vi "Buffer-GUI-parameter-values.vi"(8 "error in":errorcluster, 10 "UI ref. in":refnum<data-value>, 11 "Data ref. in":refnum<data-value>) -> (0 "error IO":errorcluster, 2 "UI ref.":refnum<data-value>, 3 "Data ref.":refnum<data-value>)   [LabVIEW 2013, in "CameraVision.lvlib" / "CV-Main.lvclass"]
doc: "This function copies the current values of the GUI parameter controls to the parameter group objects, by using the front panel object control references and the parameter group data value references."
uses:
  CV-Main.lvclass
  UI/CV-UI.lvclass
  UI/CV-UI.lvclass/CV-UI.ctl
  Configuration/Configuration-parameters-gui.ctl
  CV-Main.lvclass/CV-Main.ctl
  Acquisition/Acquisition-parameters-gui.ctl
  Acquisition/Trigger-modes.ctl
  Acquisition/Exposure-modes.ctl
  Correction/Correction-parameters-gui.ctl
  Correction/Smoothing.ctl
  Correction/Background-correction.ctl
  Analysis/Analysis-parameters-gui.ctl
  Temperature/Temperature-parameters-gui.ctl
  Mapping/Mapping-parameters-gui.ctl
  Mapping/Mapping-characteristic.ctl
  Storage/Storage-parameters-gui.ctl
  Storage/Storage-types.ctl
  Filter/Filter-parameters-gui.ctl
  Filter/Filter-settings.ctl
  Filter/Filter-characteristic.ctl
  Filter/Filter-apply.ctl
  Read Config params.vi
  Read Acquis params.vi
  Read Correct params.vi
  Read Analysis params.vi
  Read Temperature params.vi
  Read Mapping params.vi
  Read Storage params.vi
  Read Filter params.vi
  UI/Read Parameter refs.vi
  Configuration/CV-Configuration.lvclass
  Acquisition/CV-Acquisition.lvclass
  Correction/CV-Correction.lvclass
  Analysis/CV-Analysis.lvclass
  Temperature/CV-Temperature.lvclass
  Mapping/CV-Mapping.lvclass
  Storage/CV-Storage.lvclass
  Filter/CV-Filter.lvclass
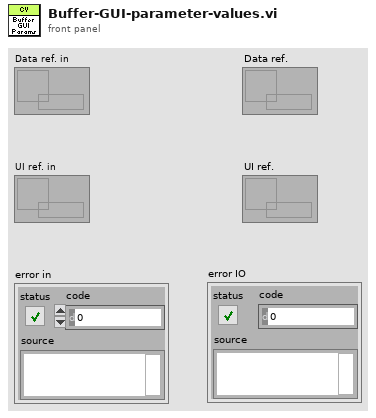
[diagram p1: front panel]
types:
  T1 = typedef "CameraVision.lvlib/CV-Configuration.lvclass/Configuration-parameters-gui.ctl" = cluster{"Number of cameras":i32, "Camera 1 port":enum16{"A", "B"}, "ROI width":u32, "ROI height":u32, "Reset ROI":bool, "Width scale":dbl, "Height scale":dbl, "Center Y cam. 1":i32, "Center X cam. 1":i32, "Center Y cam. 2":i32, "Center X cam. 2":i32}
  T2 = typedef "CameraVision.lvlib/CV-Acquisition.lvclass/Acquisition-parameters-gui.ctl" = cluster{"Acquisition mode":enum16{"Continuous", "Continuous batch", "Single batch", "Single batch -delayed"}, "Batch size":i32, "Image buffer size":i32, "Trigger mode":T3, "Duration HH":sgl, "Acquisition start":enum16{"Immediate", "Post-phoned"}, "Duration SS":sgl, "Duration MM":sgl, "Start time":timestamp, "Max. frame rate":dbl, "Exposure time cam. 1":dbl, "Exposure time cam. 2":dbl, "Exposure mode":T4, "Value 1":dbl, "Value 2":dbl, "Time 1":dbl, "Time 2":dbl}
  T3 = typedef "CameraVision.lvlib/CV-Acquisition.lvclass/Trigger-modes.ctl" = enum16{"Camera timed (not sync.)", "Framegrabber timed (sync.)", "Software timed (sync.)", "External timing (sync.)", "Manual (sync.)", "Gated - camera (not sync.)", "Gated - grabber (sync.)", "Gated - software (sync.)", "Gated - external (sync.)"}
  T4 = typedef "CameraVision.lvlib/CV-Acquisition.lvclass/Exposure-modes.ctl" = enum16{"Linear", "LinLog"}
  T5 = typedef "CameraVision.lvlib/CV-Correction.lvclass/Correction-parameters-gui.ctl" = cluster{"Background correction":bool, "Hot-pixel correction":bool, "Black image cam. 1":path, "Black image cam. 2":path, "Y-shift":i32, "X-shift":i32, "Correlation algorithm":enum16{"Fixed shift", "Cross-correlation", "Cross-correlation (5steps)", "Melt-pool center"}, "Noise treshold":sgl, "Smoothing algorithm":T6, "2nd image correlation":bool, "Image smoothing":bool, "Background correction method":T7}
  T6 = typedef "CameraVision.lvlib/CV-Correction.lvclass/Smoothing.ctl" = enum16{"Noise tresholding", "NT+Median filter", "NT+Gaussian filter"}
  T7 = typedef "CameraVision.lvlib/CV-Correction.lvclass/Background-correction.ctl" = enum16{"Hardware", "Software"}
  T8 = typedef "CameraVision.lvlib/CV-Analysis.lvclass/Analysis-parameters-gui.ctl" = cluster{"Binarization treshold":sgl, "Image characteristics":bool, "Melt-pool characteristics":bool}
  T9 = typedef "CameraVision.lvlib/CV-Temperature.lvclass/Temperature-parameters-gui.ctl" = cluster{"Temperature field":bool, "Ratio correction factor":dbl, "Temperature value":bool, "Y-coord.":dbl, "X-coord.":dbl, "Averaging center":enum16{"Fixed coordinates (pixel)", "Fixed coordinates (mm)", "Melt-pool center"}, "Averaging shape":enum16{"Point", "Circle", "Ellipse"}, "Minor axis":dbl, "Major axis":dbl}
  T10 = typedef "CameraVision.lvlib/CV-Mapping.lvclass/Mapping-parameters-gui.ctl" = cluster{"Enable mapping":bool, "Automatic timing":bool, "Scan pattern file":path, "Start off-set":dbl, "Default map characteristic":T11, "Default mark speed":i32, "Jump speed":i32}
  T11 = typedef "CameraVision.lvlib/CV-Mapping.lvclass/Mapping-characteristic.ctl" = enum16{"Average intensity [0-255]", "Peak intensity [0-255]", "Melt-pool size [mm²]", "Melt-pool aspect ratio []", "Melt-pool fragments []", "Average temperature [°C]", "Max. temperature [°C]", "Min. temperature [°C]", "Std. dev. temperature [°C]"}
  T12 = typedef "CameraVision.lvlib/CV-Storage.lvclass/Storage-parameters-gui.ctl" = cluster{"Base file name":string, "Storage directory":path, "Save what?":T13, "Image file type":enum16{"JPG", "BMP", "PNG"}, "Comments":string, "Storage mode":enum16{"1 file per layer", "1 file for all layers "}, "Start iteration/layer":u16}
  T13 = typedef "CameraVision.lvlib/CV-Storage.lvclass/Storage-types.ctl" = cluster{"Original":bool, "Corrected":bool, "Binary":bool, "Temperature":bool, "Characteristics":bool, "Mapping":bool, "TemperatureValues":bool}
  T14 = typedef "CameraVision.lvlib/CV-Filter.lvclass/Filter-parameters-gui.ctl" = cluster{"Filter array":T15[], "Storage filters":T17}
  T15 = typedef "CameraVision.lvlib/CV-Filter.lvclass/Filter-settings.ctl" = cluster{"Characteristic":T16, "Monitor":bool, "Min.":dbl, "Max.":dbl, "Min. Thres.":dbl, "Min. Dur.":u16, "Report":bool}
  T16 = typedef "CameraVision.lvlib/CV-Filter.lvclass/Filter-characteristic.ctl" = enum16{"Average intensity [0-255]", "Peak intensity [0-255]", "Melt-pool size [mm²]", "Melt-pool aspect ratio []", "Melt-pool fragments []", "Melt-pool position X [pixel]", "Melt-pool position Y [pixel]", "Average temperature [°C]", "Max. temperature [°C]", "Min. temperature [°C]", "Std. dev. temperature [°C]"}
  T17 = typedef "CameraVision.lvlib/CV-Filter.lvclass/Filter-apply.ctl" = cluster{"Filter images":bool, "Filter characteristics":bool, "Filter temperature":bool}
  T18 = typedef "CameraVision.lvlib/CV-UI.lvclass/Parameter-group-names.ctl" = enum16{"Configuration params", "Acquisition params", "Correction params", "Analysis params", "Temperature params", "Mapping params", "Storage params", "Filter params"}
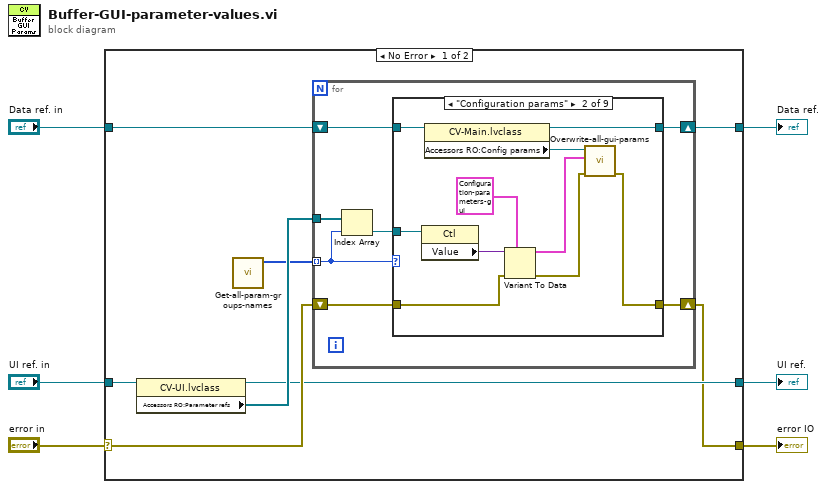
[diagram p0: block diagram]
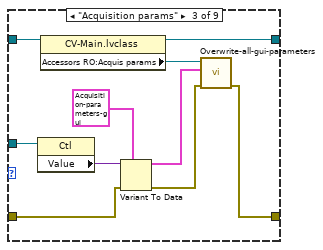
[diagram p3: hidden frame]
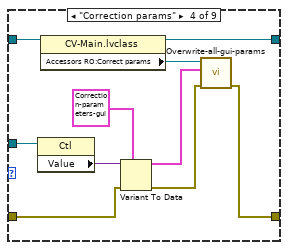
[diagram p4: hidden frame]
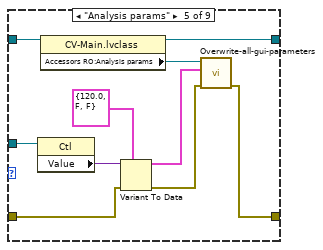
[diagram p5: hidden frame]
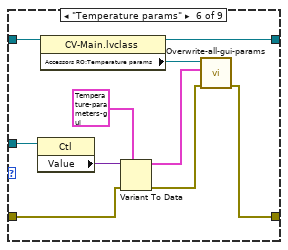
[diagram p6: hidden frame]
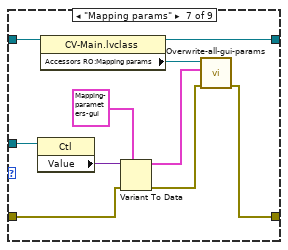
[diagram p7: hidden frame]
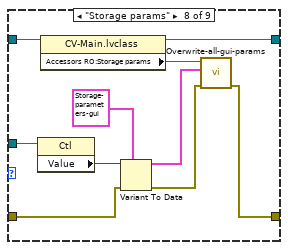
[diagram p8: hidden frame]
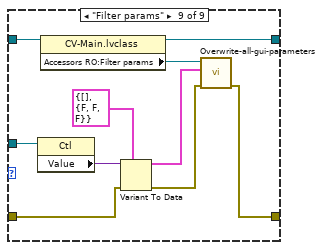
[diagram p9: hidden frame]
diagram:
  n1 = case shown="No Error" "error in" {
    selector: "error in" -> [w10 w106]
    tunnel: [w7 w106] -> w6
    tunnel: "Data ref. in" -> [w11 w105]
    tunnel: "UI ref. in" -> [w14 w104]
    tunnel: [w9 w105] -> w2
    tunnel: [w8 w104] -> w1
    frame No Error {
      n2 = property class="CV-UI.lvclass"(reference=w14) -> (reference out=w8:refnum<data-value>, "Accessors RO:Parameter refs"=w13:refnum<vi>[])  [unwired: 1 in, 1 out]
      n3 = call "Get-all-param-groups-names.vi"() -> ("Param groups"=w12:T18[])  [unwired: 11 in]
      n4 = for {
        tunnel: w12 -> [w19] mode=indexing
        tunnel: w13 -> [w21]
        shift-right: [w16] -> w7
        shift-left: w10 -> [w17]
        shift-right: [w15] -> w9
        shift-left: w11 -> [w18]
        n5 = Index Array(array=w21, index=w19) -> (element=w20:refnum<vi>)
        n6 = case shown="\"Configuration params\"" w19 {
          tunnel: w20 -> [_ w33 w43 w53 w63 w73 w83 w93 w103]
          tunnel: w18 -> [w22 w32 w42 w52 w62 w72 w82 w92 w102]
          tunnel: w17 -> [w23 w26 w39 w49 w59 w69 w79 w89 w99]
          tunnel: [w23 w25 w38 w48 w58 w68 w78 w88 w98] -> w16
          tunnel: [w22 w24 w34 w44 w54 w64 w74 w84 w94] -> w15
          frame Default {
          }
          frame "Configuration params" {
            n7 = property class="Ctl"(reference=w33) -> ("Value"=w30:variant)  [unwired: 1 in, 2 out]
            n8 = property class="CV-Main.lvclass"(reference=w32) -> (reference out=w24:refnum<data-value>, "Accessors RO:Config params"=w29:refnum<data-value>)  [unwired: 1 in, 1 out]
            n9 = Variant To Data(error in=w26, type=T1 {"Number of cameras"=1, "Camera 1 port"=enum."A", "ROI width"=1248, "ROI height"=1082, "Reset ROI"=FALSE, "Width scale"=0.05, "Height scale"=0.05, "Center Y cam. 1"=541, "Center X cam. 1"=624, "Center Y cam. 2"=541, "Center X cam. 2"=624} ("Configuration params."), Variant=w30) -> (data=w28:T1, error out=w27:errorcluster)
            n10 = call "Overwrite-all-gui-params.vi"("error in (no error)"=w27, "Configuration params."=w28, "Config. params. ref. in"=w29) -> ("error out"=w25:errorcluster)  [unwired: 7 in, 1 out]
          }
          frame "Acquisition params" {
            n11 = property class="Ctl"(reference=w43) -> ("Value"=w40:variant)  [unwired: 1 in, 2 out]
            n12 = property class="CV-Main.lvclass"(reference=w42) -> (reference out=w34:refnum<data-value>, "Accessors RO:Acquis params"=w35:refnum<data-value>)  [unwired: 1 in, 1 out]
            n13 = Variant To Data(error in=w39, type=T2 {"Acquisition mode"=enum."Continuous batch", "Batch size"=0, "Image buffer size"=1248, "Trigger mode"=enum."Gated - external (sync.)", "Duration HH"=1.0, "Acquisition start"=enum."Immediate", "Duration SS"=0.05, "Duration MM"=541.0, "Start time"=timestamp(0 s since 1904-01-01), "Max. frame rate"=541.0, "Exposure time cam. 1"=624.0, "Exposure time cam. 2"=1.0, "Exposure mode"=enum."Linear", "Value 1"=17.0, "Value 2"=14.0, "Time 1"=1000.0, "Time 2"=1000.0} ("Acquisition params."), Variant=w40) -> (data=w36:T2, error out=w37:errorcluster)
            n14 = call "Overwrite-all-gui-parameters.vi"("error in (no error)"=w37, "Acquisition params."=w36, "Acquis. params. ref. in"=w35) -> ("error out"=w38:errorcluster)  [unwired: 7 in, 1 out]
          }
          frame "Correction params" {
            n15 = property class="Ctl"(reference=w53) -> ("Value"=w50:variant)  [unwired: 1 in, 2 out]
            n16 = property class="CV-Main.lvclass"(reference=w52) -> (reference out=w44:refnum<data-value>, "Accessors RO:Correct params"=w45:refnum<data-value>)  [unwired: 1 in, 1 out]
            n17 = Variant To Data(error in=w49, type=T5 {"Background correction"=FALSE, "Hot-pixel correction"=FALSE, "Black image cam. 1"=path "C:/CameraVision/Black images/Black-CameraA-Full.bmp", "Black image cam. 2"=path "C:/CameraVision/Black images/Black-CameraB-Full.bmp", "Y-shift"=1, "X-shift"=0, "Correlation algorithm"=enum."Fixed shift", "Noise treshold"=541.0, "Smoothing algorithm"=enum."Noise tresholding", "2nd image correlation"=FALSE, "Image smoothing"=FALSE, "Background correction method"=enum."Software"} ("Correction params."), Variant=w50) -> (data=w46:T5, error out=w47:errorcluster)
            n18 = call "Overwrite-all-gui-params.vi"("error in (no error)"=w47, "Correction params."=w46, "Correct. params. ref. in"=w45) -> ("error out"=w48:errorcluster)  [unwired: 7 in, 1 out]
          }
          frame "Analysis params" {
            n19 = property class="Ctl"(reference=w63) -> ("Value"=w60:variant)  [unwired: 1 in, 2 out]
            n20 = property class="CV-Main.lvclass"(reference=w62) -> (reference out=w54:refnum<data-value>, "Accessors RO:Analysis params"=w55:refnum<data-value>)  [unwired: 1 in, 1 out]
            n21 = Variant To Data(error in=w59, type=T8 {"Binarization treshold"=120.0, "Image characteristics"=FALSE, "Melt-pool characteristics"=FALSE} ("Analys. params."), Variant=w60) -> (data=w56:T8, error out=w57:errorcluster)
            n22 = call "Overwrite-all-gui-parameters.vi"("error in (no error)"=w57, "Analys. params."=w56, "Analysis params. ref. in"=w55) -> ("error out"=w58:errorcluster)  [unwired: 7 in, 1 out]
          }
          frame "Temperature params" {
            n23 = property class="Ctl"(reference=w73) -> ("Value"=w70:variant)  [unwired: 1 in, 2 out]
            n24 = property class="CV-Main.lvclass"(reference=w72) -> (reference out=w64:refnum<data-value>, "Accessors RO:Temperature params"=w65:refnum<data-value>)  [unwired: 1 in, 1 out]
            n25 = Variant To Data(error in=w69, type=T9 {"Temperature field"=FALSE, "Ratio correction factor"=1.0, "Temperature value"=FALSE, "Y-coord."=0.0, "X-coord."=0.0, "Averaging center"=enum."Fixed coordinates (mm)", "Averaging shape"=enum."Point", "Minor axis"=0.0, "Major axis"=0.0} ("Temperature params."), Variant=w70) -> (data=w66:T9, error out=w67:errorcluster)
            n26 = call "Overwrite-all-gui-params.vi"("error in (no error)"=w67, "Temperature params."=w66, "Temp. params. ref. in"=w65) -> ("error out"=w68:errorcluster)  [unwired: 7 in, 1 out]
          }
          frame "Mapping params" {
            n27 = property class="Ctl"(reference=w83) -> ("Value"=w80:variant)  [unwired: 1 in, 2 out]
            n28 = property class="CV-Main.lvclass"(reference=w82) -> (reference out=w74:refnum<data-value>, "Accessors RO:Mapping params"=w75:refnum<data-value>)  [unwired: 1 in, 1 out]
            n29 = Variant To Data(error in=w79, type=T10 {"Enable mapping"=FALSE, "Automatic timing"=FALSE, "Scan pattern file"=path "C:/CameraVision/Scan patterns/Template.sp", "Start off-set"=0.0, "Default map characteristic"=enum."Average intensity [0-255]", "Default mark speed"=1, "Jump speed"=0} ("Temperature params."), Variant=w80) -> (data=w76:T10, error out=w77:errorcluster)
            n30 = call "Overwrite-all-gui-params.vi"("error in (no error)"=w77, "Mapping params."=w76, "Mapping params. ref. in"=w75) -> ("error out"=w78:errorcluster)  [unwired: 7 in, 1 out]
          }
          frame "Storage params" {
            n31 = property class="Ctl"(reference=w93) -> ("Value"=w90:variant)  [unwired: 1 in, 2 out]
            n32 = property class="CV-Main.lvclass"(reference=w92) -> (reference out=w84:refnum<data-value>, "Accessors RO:Storage params"=w85:refnum<data-value>)  [unwired: 1 in, 1 out]
            n33 = Variant To Data(error in=w89, type=T12 {"Base file name"="Test", "Storage directory"=path "C:/CameraVision/Results", "Save what?"={"Original"=FALSE, "Corrected"=FALSE, "Binary"=FALSE, "Temperature"=FALSE, "Characteristics"=FALSE, "Mapping"=FALSE, "TemperatureValues"=FALSE}, "Image file type"=enum."BMP", "Comments"="", "Storage mode"=enum."1 file for all layers ", "Start iteration/layer"=0} ("Temperature params."), Variant=w90) -> (data=w86:T12, error out=w87:errorcluster)
            n34 = call "Overwrite-all-gui-params.vi"("error in (no error)"=w87, "Storage params."=w86, "Storage params. ref. in"=w85) -> ("error out"=w88:errorcluster)  [unwired: 7 in, 1 out]
          }
          frame "Filter params" {
            n35 = property class="Ctl"(reference=w103) -> ("Value"=w100:variant)  [unwired: 1 in, 2 out]
            n36 = property class="CV-Main.lvclass"(reference=w102) -> (reference out=w94:refnum<data-value>, "Accessors RO:Filter params"=w95:refnum<data-value>)  [unwired: 1 in, 1 out]
            n37 = Variant To Data(error in=w99, type=T14 {"Filter array"=[], "Storage filters"={"Filter images"=FALSE, "Filter characteristics"=FALSE, "Filter temperature"=FALSE}} ("Temperature params."), Variant=w100) -> (data=w96:T14, error out=w97:errorcluster)
            n38 = call "Overwrite-all-gui-parameters.vi"("error in (no error)"=w97, "Filter params."=w96, "Filter params. ref. in"=w95) -> ("error out"=w98:errorcluster)  [unwired: 7 in, 1 out]
          }
        }
      }
    }
    frame Error {
    }
  }
  "error IO" <- w6
  "Data ref." <- w2
  "UI ref." <- w1
